vi "Config dialog.vi"(8 "error in (no error)":errorcluster, 10 "Mono config":T2={"VISA resource "="", "nm/min"=100.0}, 11 "Lock-in config":T1) -> (0 "error out":errorcluster, 1 "Cancelled?":bool, 2 "Mono config out":T2={"VISA resource "="", "nm/min"=100.0}, 3 "Lock-in config out":T1)   [LabVIEW 2020]
uses:
  controls/Config dialog states.ctl
  controls/Lock-in config.ctl
  controls/Mono config.ctl
panel:
  out "Lock-in config (old)":T1
  out "Mono config (old)":T2={"VISA resource "="", "nm/min"=100.0}
  in  "OK":bool
  in  "Cancel":bool
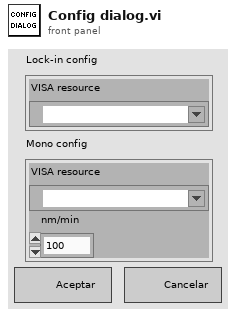
[diagram p1: front panel]
types:
  T1 = typedef "Lock-in config.ctl" = cluster{"VISA resource ":refnum<visa-resource-name>}
  T2 = typedef "Mono config.ctl" = cluster{"VISA resource ":refnum<visa-resource-name>, "nm/min":dbl}
  T3 = typedef "Config dialog states.ctl" = enum16{"Initialize", "Update values", "Wait", "Exit", "Cancel"}
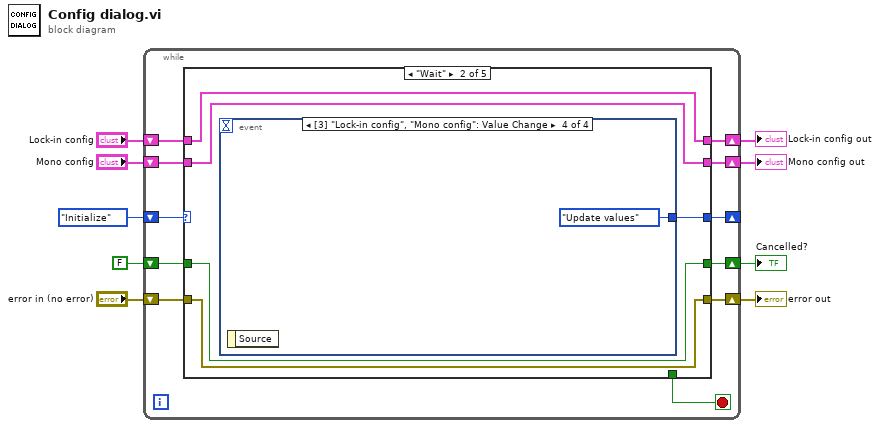
[diagram p0: block diagram]
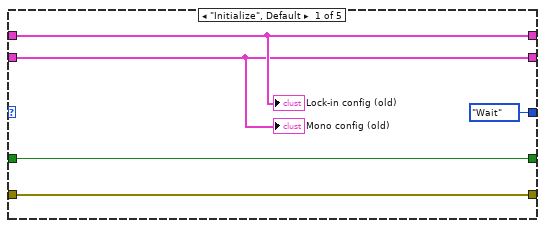
[diagram p2: hidden frame]
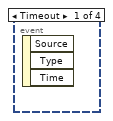
[diagram p3: hidden frame]
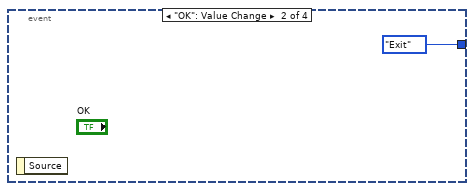
[diagram p4: hidden frame]
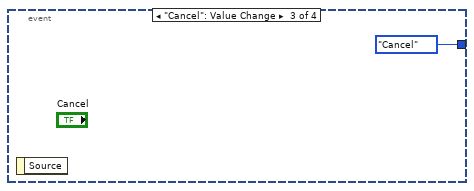
[diagram p5: hidden frame]
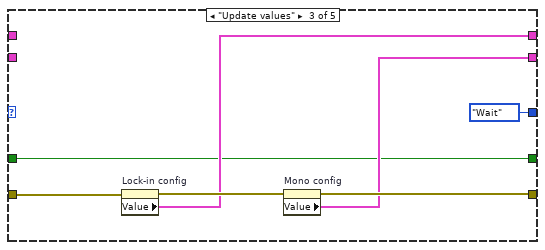
[diagram p6: hidden frame]
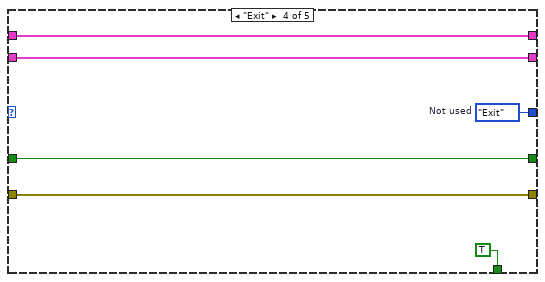
[diagram p7: hidden frame]
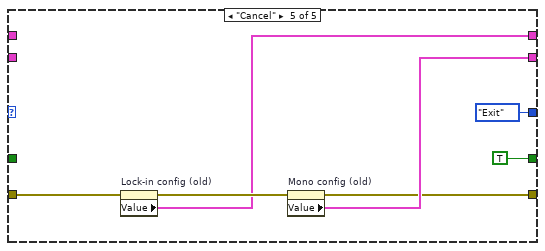
[diagram p8: hidden frame]
diagram:
  n1 = while {
    shift-right: [w19] -> _
    shift-left: Config_dialog_states."Initialize" -> [w20]
    shift-right: [w16] -> w7
    shift-left: "error in (no error)" -> [w17]
    shift-right: [w13] -> w4
    shift-left: "Lock-in config" -> [w14]
    shift-right: [w12] -> w3
    shift-left: "Mono config" -> [w15]
    shift-right: [w11] -> w2
    shift-left: FALSE -> [w10]
    stop <- w18 stop-if-true
    n2 = case shown="\"Wait\"" w20 {
      tunnel: [Config_dialog_states."Wait" w30 Config_dialog_states."Wait" w45 Config_dialog_states."Exit"] -> w19
      tunnel: [_ _ _ TRUE _] -> w18
      tunnel: w17 -> [w24 w29 w40 w44 w51]
      tunnel: [w24 w29 w38 w44 w49] -> w16
      tunnel: w15 -> [w22 w27 _ w42 _]
      tunnel: w14 -> [w23 w28 _ w43 _]
      tunnel: [w23 w28 w37 w43 w48] -> w13
      tunnel: [w22 w27 w36 w42 w52] -> w12
      tunnel: [w21 w26 w34 w41 TRUE] -> w11
      tunnel: w10 -> [w21 w26 w34 w41 _]
      frame "Initialize", Default {
        "Lock-in config (old)" <- w23
        "Mono config (old)" <- w22
      }
      frame "Wait" {
        n3 = event shown="[3] \"Lock-in config\", \"Mono config\": Value Change" {
          selector: _ -> [_ _ _ _]
          dyn-events: _ -> [_ _ _ _]
          timeout: _ -> [_ _ _ _]
          tunnel: [_ Config_dialog_states."Exit" Config_dialog_states."Cancel" Config_dialog_states."Update values"] -> w30
          event Timeout {
            n4 = event-data() -> ()  [unwired: 1 in, 3 out]
          }
          event "OK": Value Change {
            n5 = event-data() -> ()  [unwired: 1 in, 1 out]
          }
          event "Cancel": Value Change {
            n6 = event-data() -> ()  [unwired: 1 in, 1 out]
          }
          event Value Change {
            n7 = event-data() -> ()  [unwired: 1 in, 1 out]
          }
        }
      }
      frame "Update values" {
        n8 = property on="Lock-in config" class="Clust (strict)"(error in=w40) -> (error out=w39:errorcluster, "Value"=w37:T1)  [unwired: 1 in, 1 out]
        n9 = property on="Mono config" class="Clust (strict)"(error in=w39) -> (error out=w38:errorcluster, "Value"=w36:T2)  [unwired: 1 in, 1 out]
      }
      frame "Exit" {
        w45 = Config_dialog_states."Exit"  # Not used
      }
      frame "Cancel" {
        n10 = property on="Lock-in config (old)" class="Clust (strict)"(error in=w51) -> (error out=w50:errorcluster, "Value"=w48:T1)  [unwired: 1 in, 1 out]
        n11 = property on="Mono config (old)" class="Clust (strict)"(error in=w50) -> (error out=w49:errorcluster, "Value"=w52:T2)  [unwired: 1 in, 1 out]
      }
    }
  }
  "Lock-in config out" <- w4
  "Mono config out" <- w3
  "error out" <- w7
  "Cancelled?" <- w2
